vi "3d_display5.vi"() -> ()   [LabVIEW 2009]
doc: "This example demonstrates some fundamental concepts for the 3D picture control. Concepts covered include:\n\n-Object creation\n-Texturing\n-Object movement\n-Object hierarchy"
uses:
  labWOOOO/wiimotestate.ctl
  labWOOOO/wiimoteState(IR).ctl
  <vilib>/Utility/miscctls.llb/LVRectTypeDef.ctl
  C:/Documents and Settings/pbooth/My Documents/labWOOOO/WiimoteLib.dll
  <vilib>/picture/3D Picture Control/NI_3D Picture Control.lvlib
  <vilib>/Analysis/NI_AALBase.lvlib
panel:
  out "angle":dbl
  in  "Y":dbl
  out "trackerino":bool
  out "Blinky":bool
  out "angle 3":sgl
  out "Value 2":sgl
  out "Value":sgl
  out "Cluster":cluster{"Wiimote State":T1, "IRState":T2} {"IRState"."Mode" items=["Off"=0, "Basic"=1, "Extended"=3, "Full"=5]}
  out "raw pitot":dbl
  in  "Calibrate pitot":bool
  in  "voltage offset":dbl=2.5
  in  "velocity scale":dbl=100000.0
  in  "Set Start Time (s)":dbl
  in  "X":dbl
  in  "Z":dbl
  in  "Calibrate Z":bool
  in  "Calibrate Y":bool
  in  "Calibrate X":bool
  out "angle 2":dbl
  out "angle 1":dbl
  out "X mean acceleration":dbl format="%0.4f"
  out "Y mean acceleration":dbl format="%0.4f"
  out "X mean volts":dbl format="%0.4f"
  out "Y mean volts":dbl format="%0.4f"
  out "Z mean acceleration":dbl format="%0.4f"
  out "Z mean volts":dbl format="%0.4f"
  in  "z gain":dbl=5.0
  in  "z offset":dbl=1.25
  in  "y gain":dbl=5.0
  in  "y offset":dbl=1.25
  in  "x gain":dbl=5.0
  in  "x offset":dbl=1.25
  in  "Render Dest":enum16{"Scene Window", "Scene Display"}(ring)=enum."Scene Display"
  in  "Camera Controller":enum16{"None", "Spherical", "Flying"}(ring)=enum."Spherical"
  out "Scene Display":refnum<vi>(3d-picture)
  in  "stop":bool
  # "Accelerometers"
  # "Buttons"
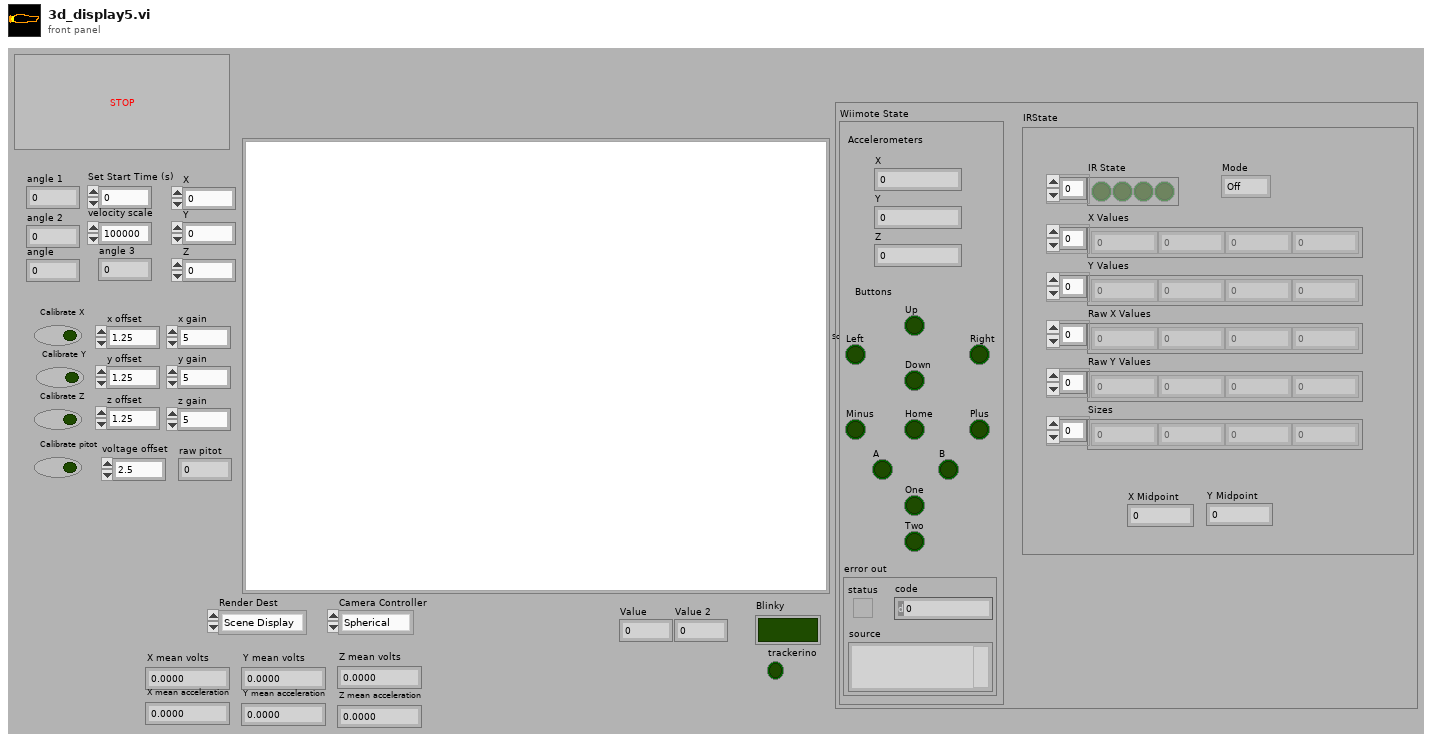
[diagram p1: front panel]
types:
  T1 = typedef "wiimotestate.ctl" = cluster{"X":sgl, "Y":sgl, "Z":sgl, "A":bool, "B":bool, "Down":bool, "Home":bool, "Left":bool, "Minus":bool, "One":bool, "Plus":bool, "Right":bool, "Two":bool, "Up":bool, "error out":errorcluster}
  T2 = typedef "wiimoteState(IR).ctl" = cluster{"Mode":u8, "IR State":bool[], "X Values":sgl[], "Y Values":sgl[], "Raw X Values":i32[], "Raw Y Values":i32[], "Sizes":i32[], "X Midpoint":sgl, "Y Midpoint":sgl}
  T3 = enum16{"As a Decal", "With Modulation", "With Blending", "As a replacement"}
  T4 = typedef "LVRectTypeDef.ctl" = cluster{"Left":i16, "Top":i16, "Right":i16, "Bottom":i16}
  T5 = enum16{"Open", "Minimized", "Maximized", "Hidden"}
  T6 = typedef "imagedata.ctl" = cluster{"image type":i32, "image depth":i32, "image":u8[], "mask":u8[], "colors":u32[], "Rectangle":cluster{"left":i16, "top":i16, "right":i16, "bottom":i16}}
  T7 = cluster{"Mode":u8, "IR State":bool[], "X Values":sgl[], "Y Values":sgl[], "Raw X Values":i32[], "Raw Y Values":i32[], "Sizes":i32[], "X Midpoint":sgl, "Y Midpoint":sgl}
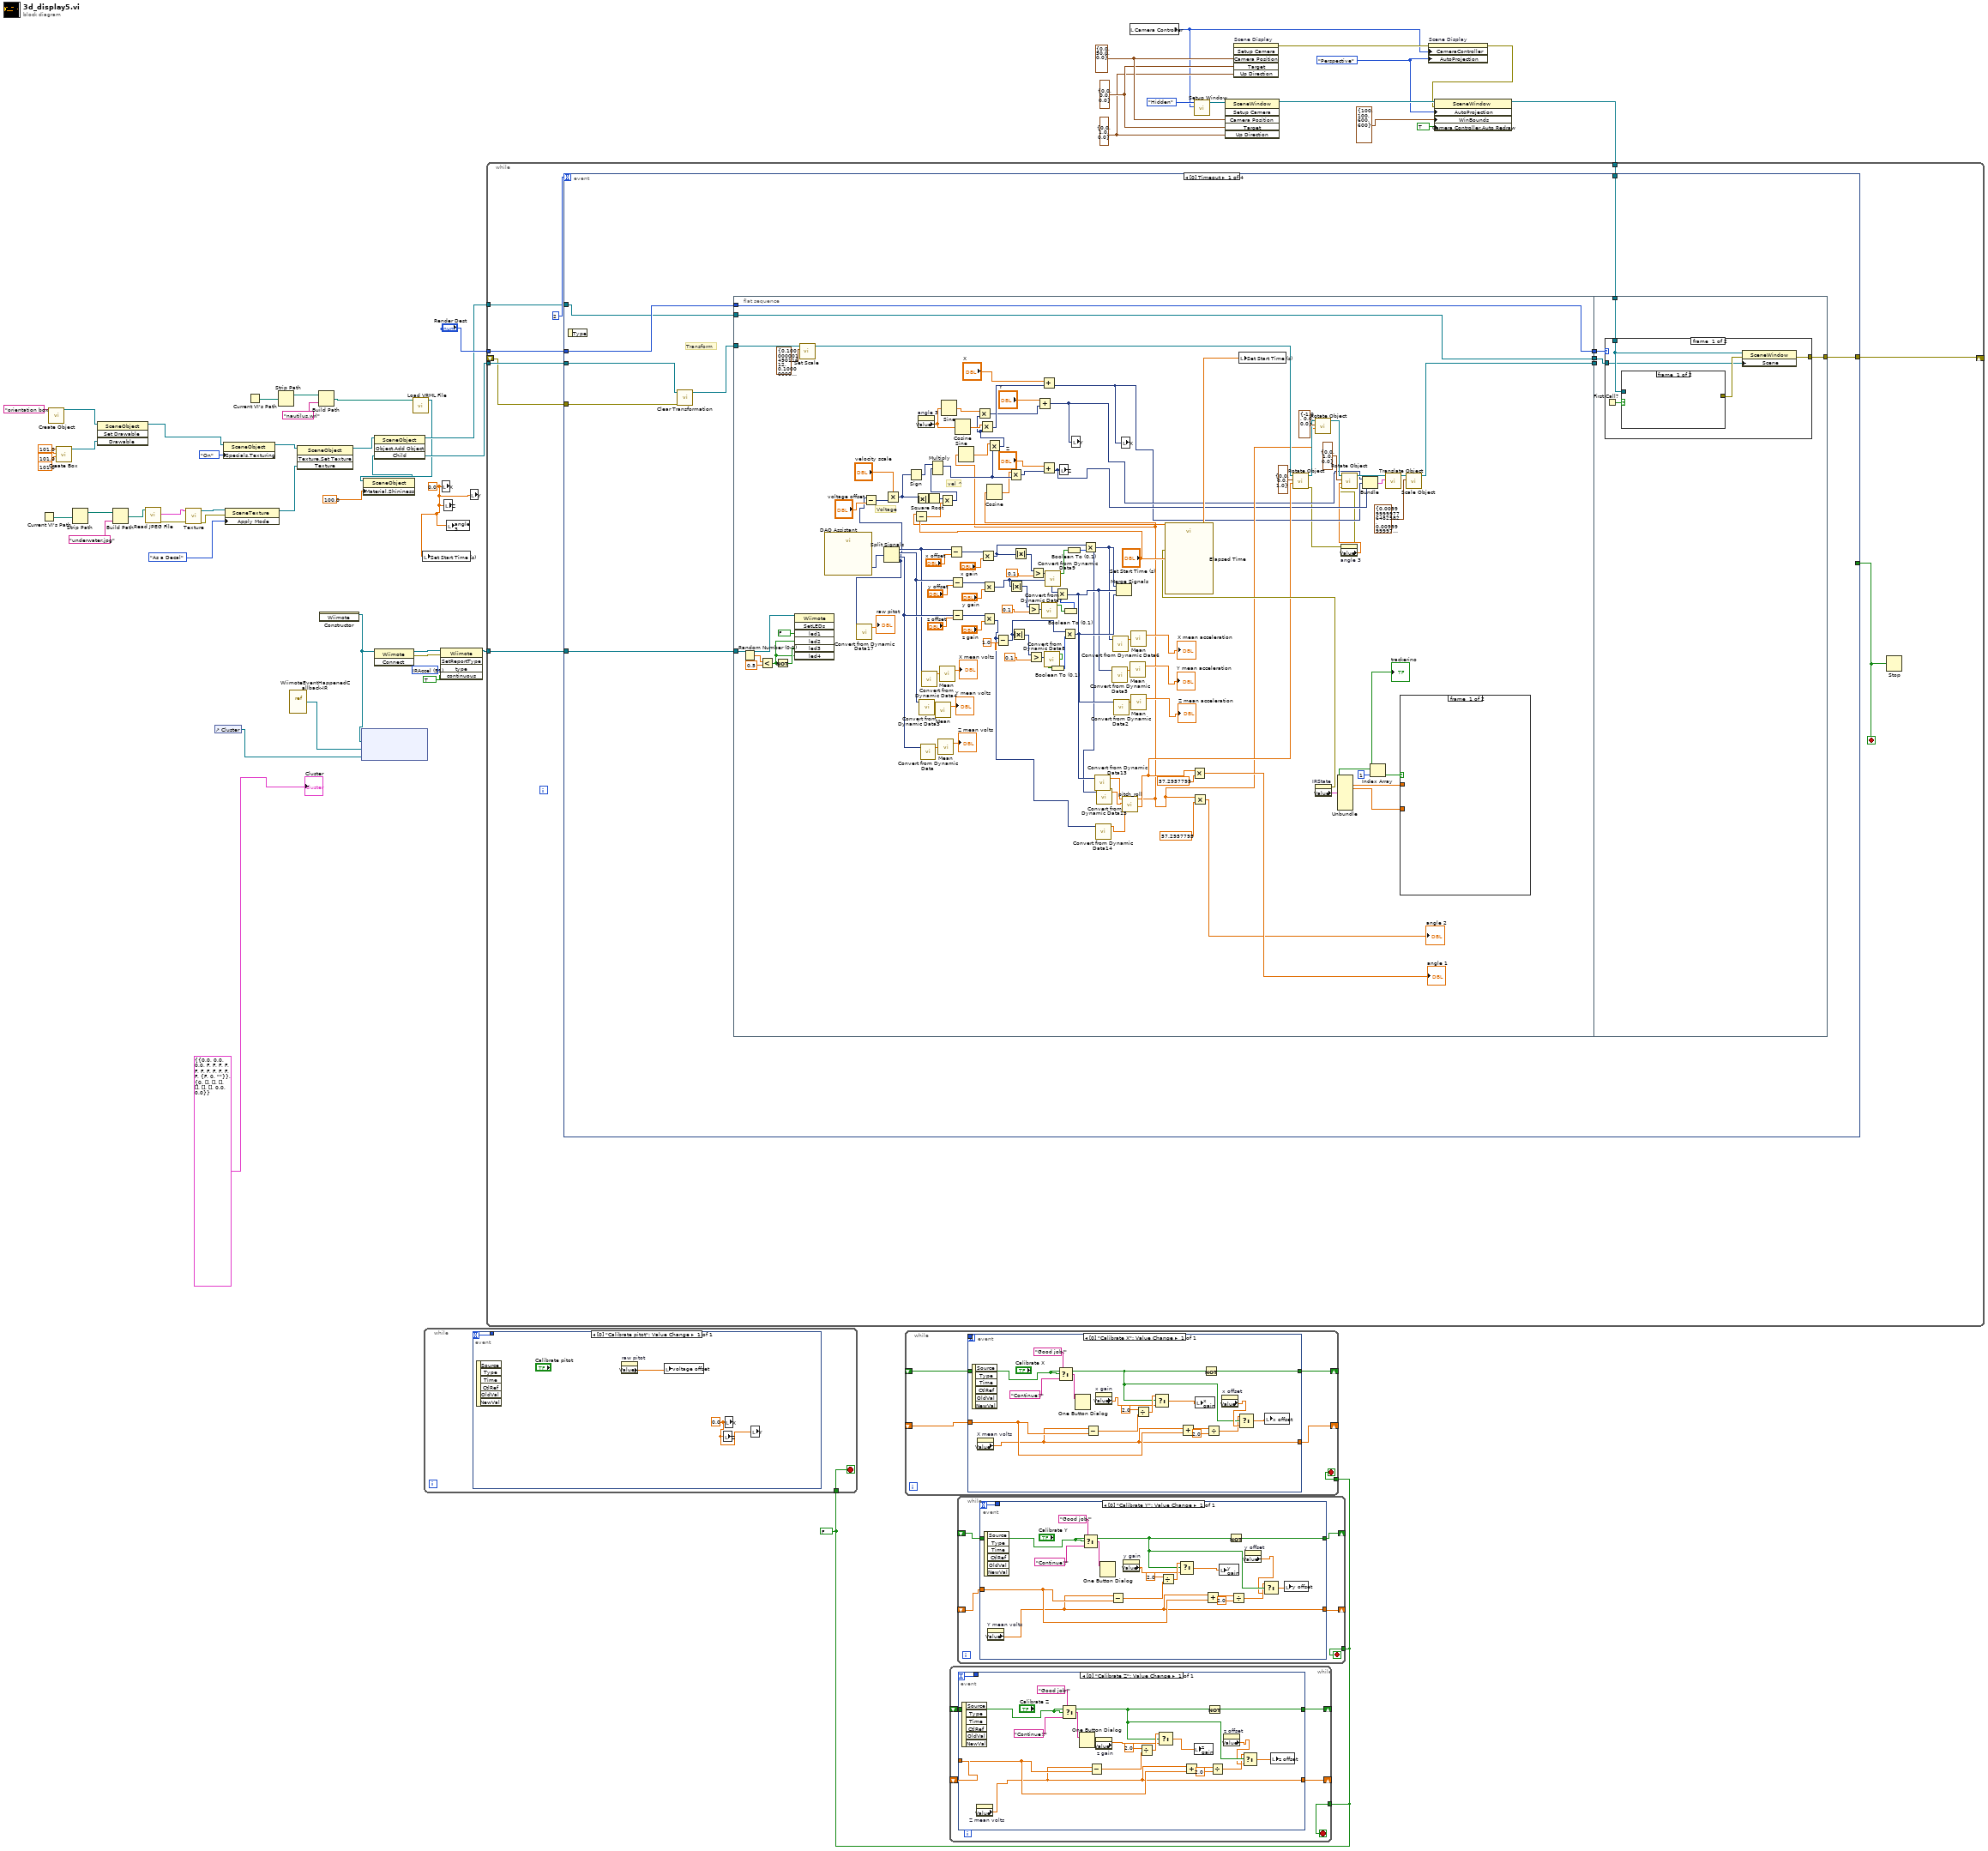
[diagram p0: block diagram]
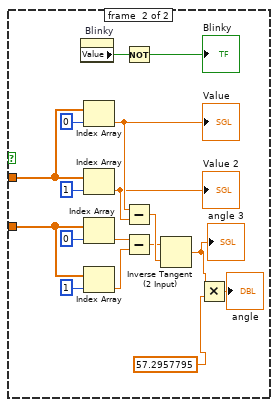
[diagram p2: hidden frame]
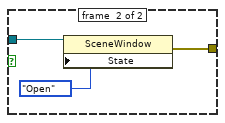
[diagram p3: hidden frame]
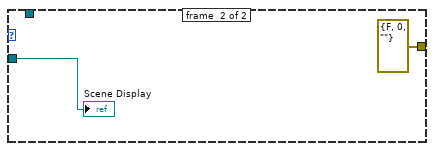
[diagram p4: hidden frame]
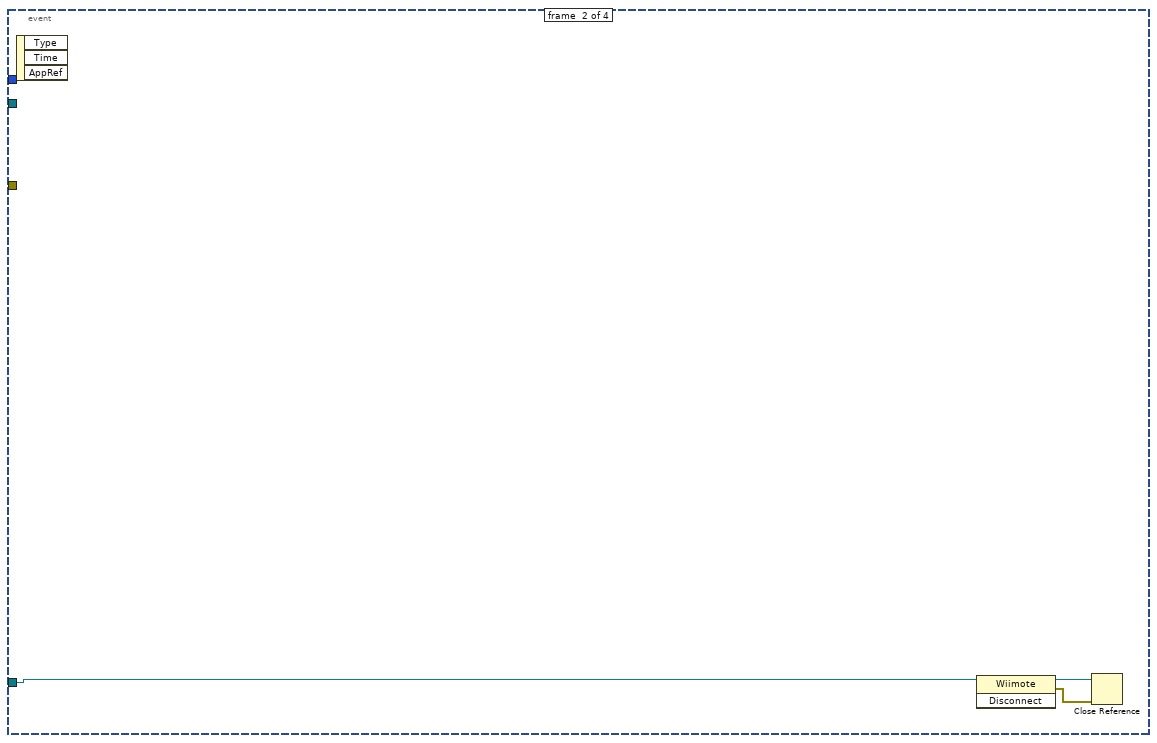
[diagram p5: hidden frame]
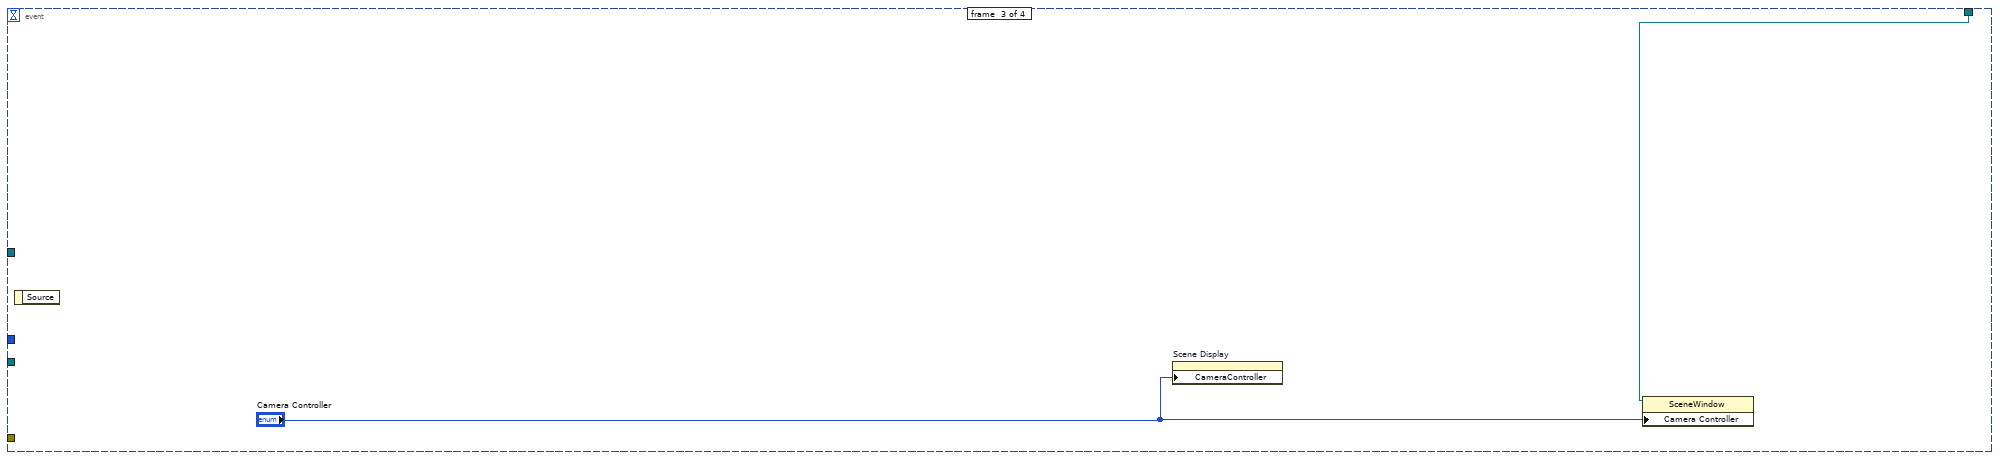
[diagram p6: hidden frame]
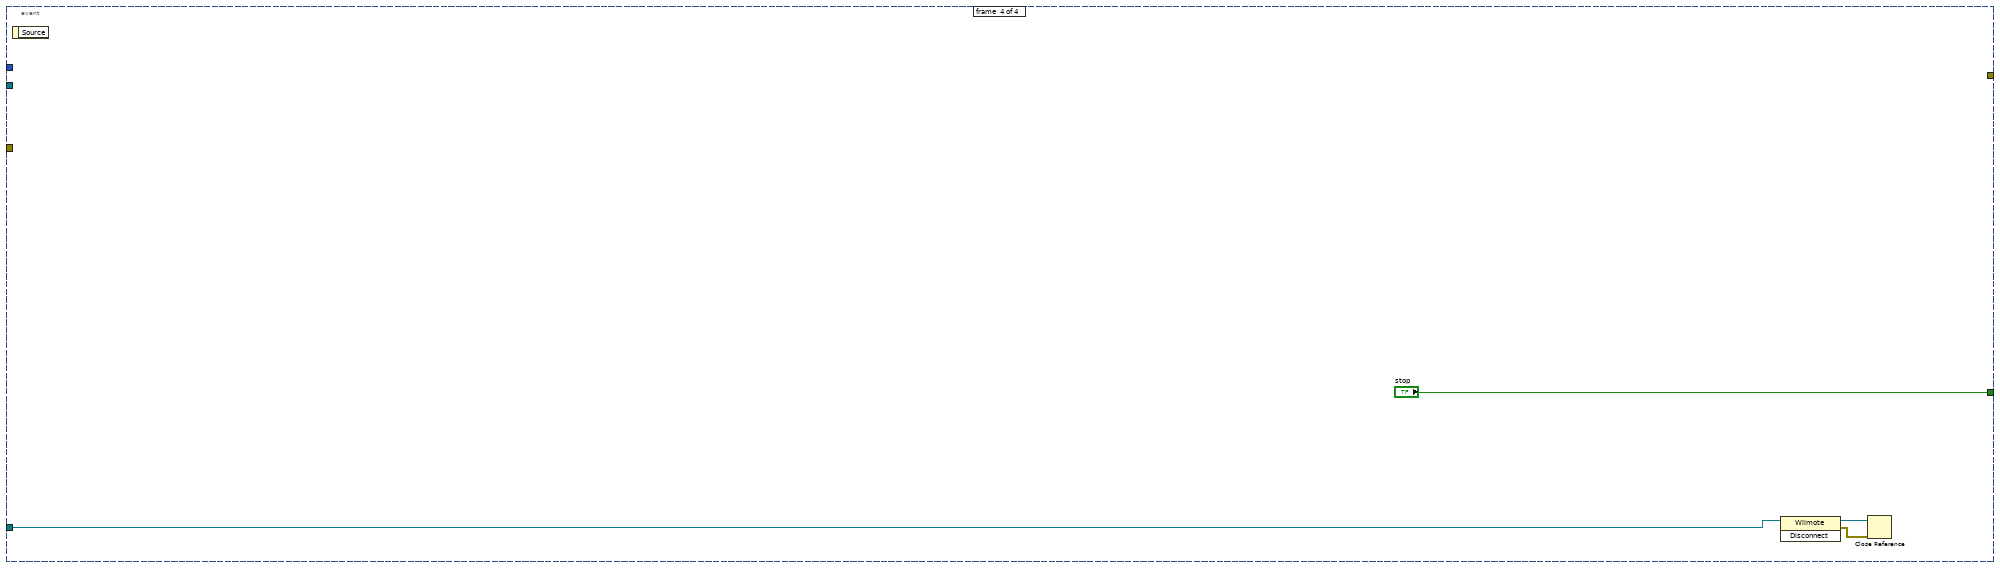
[diagram p7: hidden frame]
diagram:
  w7 = FALSE
  w32 = u8 51 items=["Status"=32, "ReadData"=33, "Buttons"=48, "ButtonsAccel"=49, "IRAccel"=51, "ButtonsExtension"=52, "ExtensionAccel"=53, "IRExtensionAccel"=55] ("type")
  w9 = 0.0 ("X")
  w48 = enum16{"None", "Perspective", "Orthographic"}."Perspective" ("Auto Projection Mode")
  w51 = cluster{"X":sgl, "Y":sgl, "Z":sgl} {"X"=0.0, "Y"=1.0, "Z"=0.0} ("Up Direction")
  w52 = cluster{"X":sgl, "Y":sgl, "Z":sgl} {"X"=0.0, "Y"=0.0, "Z"=0.0} ("Target")
  w53 = cluster{"X":sgl, "Y":sgl, "Z":sgl} {"X"=0.0, "Y"=50.0, "Z"=0.0} ("Camera Position")
  n1 = Current VI's Path() -> (path=w22:path)
  n2 = call <vilib>:"Create Object.vi"("Name"="orientation box") -> ("Scene:New Object"=w26:refnum<vi>)  [unwired: 9 in, 1 out]
  n3 = call <vilib>:"Create Box.vi"("Length Z"=sgl 101.0, "Length Y"=sgl 101.0, "Length X"=sgl 101.0) -> ("New Box Refnum"=w24:refnum<vi>)  [unwired: 7 in, 1 out]
  n4 = Strip Path(path=w22) -> (stripped path=w23:path)  [unwired: 1 out]
  n5 = invoke class="SceneObject" method="Set Drawable"(reference=w26, "Drawable"=w24) -> (reference out=w15:refnum<vi>)  [unwired: 2 in, 3 out]
  n6 = Build Path(base path=w23, name or relative path="underwater.jpg") -> (appended path=w20:path)
  n7 = call <vilib>:"Read JPEG File.vi"("path to JPEG file"=w20) -> ("error out"=w13:errorcluster, "image data"=w14:T6)  [unwired: 8 in, 1 out]
  n8 = call <vilib>:"Texture.vi"("error in (no error)"=w13, "Image"=w14) -> ("error out"=w12:errorcluster, "New Texture Refnum"=w11:refnum<vi>)  [unwired: 8 in]
  n9 = control-ref of="Cluster"() -> (w35:refnum<vi>)
  n10 = property class="SceneObject"(reference=w15, "Specials.Texturing"=enum16{"Inherit Value", "Off", "On"}."On" ("Specials:Texturing")) -> (reference out=w16:refnum<vi>)  [unwired: 1 in, 1 out]
  n11 = property class="SceneTexture"(reference=w11, error in=w12, "Apply Mode"=T3."As a Decal") -> (reference out=w18:refnum<vi>)  [unwired: 1 out]
  n12 = Current VI's Path() -> (path=w41:path)
  n13 = Strip Path(path=w41) -> (stripped path=w42:path)  [unwired: 1 out]
  n14 = vi-ref "WiimoteEventHappenedCallback-IR.vi"() -> ("vi reference"=w38:refnum<vi>)
  n15 = invoke class="SceneObject" method="Texture.Set Texture"(reference=w16, "Texture"=w18) -> (reference out=w6:refnum<vi>)  [unwired: 2 in, 3 out]
  n16 = Build Path(base path=w42, name or relative path="nautilus.wrl") -> (appended path=w39:path)
  n17 = constructor class="Wiimote"() -> (reference out=w37:refnum<k24>)  [unwired: 3 in, 2 out]
  n18 = node(w37, w38, w35) -> ()  [unwired: 2 in, 2 out]
  n19 = invoke class="Wiimote" method="Connect"(reference=w37) -> (reference out=w34:refnum<k24>, error out=w33:errorcluster)  [unwired: 2 in, 1 out]
  n20 = call <vilib>:"Load VRML File.vi"("Path"=w39) -> ("Scene:Read Scene File"=w2:refnum<vi>)  [unwired: 9 in, 1 out]
  n21 = property class="SceneObject"(reference=w2, "Material.Shininess"=sgl 100.0 ("Material:Shininess")) -> (reference out=w1:refnum<vi>)  [unwired: 1 in, 1 out]
  n22 = invoke class="SceneObject" method="Object.Add Object"(reference=w6, "Child"=w1) -> (reference out=w4:refnum<vi>, "Child"=w5:refnum<vi>)  [unwired: 2 in, 2 out]
  n23 = local write "Set Start Time (s)"(w9) -> ()
  n24 = while {
    tunnel: w7 -> [w55]
    stop <- w55 stop-if-true
    n25 = event shown="[0] \"Calibrate pitot\": Value Change" {
      selector: _ -> [_]
      dyn-events: _ -> [_]
      timeout: _ -> [w58]
      tunnel: [w58] -> _
      event [0] "Calibrate pitot": Value Change {
        w56 = 0.0 ("X")
        n26 = event-data() -> ()  [unwired: 1 in, 6 out]
        n27 = property on="raw pitot" class="DigNum (strict)"() -> ("Value"=w57:dbl)  [unwired: 2 in, 2 out]
        n28 = local write "voltage offset"(w57) -> ()
        n29 = local write "Z"(w56) -> ()
        n30 = local write "X"(w56) -> ()
        n31 = local write "Y"(w56) -> ()
      }
    }
  }
  n32 = invoke class="Wiimote" method="SetReportType"(reference=w34, error in=w33, "type"=w32, "continuous"=TRUE) -> (reference out=w8:refnum<k24>)  [unwired: 1 in, 4 out]
  n33 = local write "X"(w9) -> ()
  n34 = local write "Z"(w9) -> ()
  n35 = local write "angle 3"(w9) -> ()
  n36 = local write "Y"(w9) -> ()
  n37 = while {
    shift-right: [w62] -> _
    shift-left: _ -> [w63]
    shift-right: [w61] -> _
    shift-left: _ -> [w60]
    tunnel: w7 -> [w59]
    stop <- w59 stop-if-true
    n38 = event shown="[0] \"Calibrate X\": Value Change" {
      selector: _ -> [_]
      dyn-events: _ -> [_]
      timeout: _ -> [w81]
      tunnel: [w81] -> _
      tunnel: w63 -> [w69]
      tunnel: [w77] -> w62
      tunnel: [w64] -> w61
      tunnel: w60 -> [w68]
      event [0] "Calibrate X": Value Change {
        n39 = event-data() -> ()  [unwired: 1 in, 6 out]
        n40 = property on="X mean volts" class="DigNum (strict)"() -> ("Value"=w64:dbl)  [unwired: 2 in, 2 out]
        n41 = Select(t="Good job!" ("message"), s=w69, f="Continue!!" ("message")) -> (s? t:f=w80:string)
        n42 = One Button Dialog(message=w80) -> ()  [unwired: 1 in, 1 out]
        n43 = Subtract(x=w64, y=w68) -> (x-y=w75:dbl)
        n44 = property on="x gain" class="DigNum (strict)"() -> ("Value"=w73:dbl)  [unwired: 2 in, 2 out]
        n45 = Divide(x=2.0, y=w75) -> (x/y=w74:dbl)
        n46 = Select(t=w74, s=w69, f=w73) -> (s? t:f=w72:dbl)
        n47 = Add(x=w64, y=w68) -> (x+y=w66:dbl)
        n48 = local write "x gain"(w72) -> ()
        n49 = Not(x=w69) -> (.not. x?=w77:bool)
        n50 = Divide(x=w66, y=2.0) -> (x/y=w65:dbl)
        n51 = property on="x offset" class="DigNum (strict)"() -> ("Value"=w70:dbl)  [unwired: 2 in, 2 out]
        n52 = Select(t=w65, s=w69, f=w70) -> (s? t:f=w71:dbl)
        n53 = local write "x offset"(w71) -> ()
      }
    }
  }
  n54 = while {
    shift-right: [w84] -> _
    shift-left: _ -> [w83]
    shift-right: [w86] -> _
    shift-left: _ -> [w85]
    tunnel: w7 -> [w82]
    stop <- w82 stop-if-true
    n55 = event shown="[0] \"Calibrate Z\": Value Change" {
      selector: _ -> [_]
      dyn-events: _ -> [_]
      timeout: _ -> [w104]
      tunnel: [w104] -> _
      tunnel: w85 -> [w96]
      tunnel: [w100] -> w86
      tunnel: [w87] -> w84
      tunnel: w83 -> [w95]
      event [0] "Calibrate Z": Value Change {
        n56 = event-data() -> ()  [unwired: 1 in, 6 out]
        n57 = property on="Z mean volts" class="DigNum (strict)"() -> ("Value"=w87:dbl)  [unwired: 2 in, 2 out]
        n58 = Select(t="Good job!" ("message"), s=w96, f="Continue!!" ("message")) -> (s? t:f=w103:string)
        n59 = One Button Dialog(message=w103) -> ()  [unwired: 1 in, 1 out]
        n60 = Subtract(x=w87, y=w95) -> (x-y=w98:dbl)
        n61 = property on="z gain" class="DigNum (strict)"() -> ("Value"=w90:dbl)  [unwired: 2 in, 2 out]
        n62 = Divide(x=2.0, y=w98) -> (x/y=w97:dbl)
        n63 = Select(t=w97, s=w96, f=w90) -> (s? t:f=w88:dbl)
        n64 = Add(x=w87, y=w95) -> (x+y=w93:dbl)
        n65 = local write "z gain"(w88) -> ()
        n66 = Not(x=w96) -> (.not. x?=w100:bool)
        n67 = Divide(x=w93, y=2.0) -> (x/y=w92:dbl)
        n68 = property on="z offset" class="DigNum (strict)"() -> ("Value"=w89:dbl)  [unwired: 2 in, 2 out]
        n69 = Select(t=w92, s=w96, f=w89) -> (s? t:f=w91:dbl)
        n70 = local write "z offset"(w91) -> ()
      }
    }
  }
  n71 = while {
    shift-right: [w109] -> _
    shift-left: _ -> [w108]
    shift-right: [w106] -> _
    shift-left: _ -> [w107]
    tunnel: w7 -> [w105]
    stop <- w105 stop-if-true
    n72 = event shown="[0] \"Calibrate Y\": Value Change" {
      selector: _ -> [_]
      dyn-events: _ -> [_]
      timeout: _ -> [w127]
      tunnel: [w127] -> _
      tunnel: w108 -> [w119]
      tunnel: [w123] -> w109
      tunnel: [w110] -> w106
      tunnel: w107 -> [w118]
      event [0] "Calibrate Y": Value Change {
        n73 = event-data() -> ()  [unwired: 1 in, 6 out]
        n74 = property on="Y mean volts" class="DigNum (strict)"() -> ("Value"=w110:dbl)  [unwired: 2 in, 2 out]
        n75 = Select(t="Good job!" ("message"), s=w119, f="Continue!!" ("message")) -> (s? t:f=w126:string)
        n76 = One Button Dialog(message=w126) -> ()  [unwired: 1 in, 1 out]
        n77 = Subtract(x=w110, y=w118) -> (x-y=w121:dbl)
        n78 = property on="y gain" class="DigNum (strict)"() -> ("Value"=w114:dbl)  [unwired: 2 in, 2 out]
        n79 = Divide(x=2.0, y=w121) -> (x/y=w120:dbl)
        n80 = Select(t=w120, s=w119, f=w114) -> (s? t:f=w113:dbl)
        n81 = Add(x=w110, y=w118) -> (x+y=w116:dbl)
        n82 = local write "y gain"(w113) -> ()
        n83 = Not(x=w119) -> (.not. x?=w123:bool)
        n84 = Divide(x=w116, y=2.0) -> (x/y=w115:dbl)
        n85 = property on="y offset" class="DigNum (strict)"() -> ("Value"=w112:dbl)  [unwired: 2 in, 2 out]
        n86 = Select(t=w115, s=w119, f=w112) -> (s? t:f=w111:dbl)
        n87 = local write "y offset"(w111) -> ()
      }
    }
  }
  n88 = local read "Camera Controller"() -> (w45:enum16{"None", "Spherical", "Flying"})
  n89 = call <vilib>:"Setup Window.vi"("Camera Controller"=w45, "Window State"=T5."Hidden") -> ("New Window Refnum"=w47:refnum<vi>)  [unwired: 1 in, 8 out]
  n90 = invoke class="SceneWindow" method="Setup Camera"(reference=w47, "Camera Position"=w53, "Target"=w52, "Up Direction"=w51) -> (reference out=w54:refnum<vi>)  [unwired: 2 in, 5 out]
  n91 = invoke on="Scene Display" class="SceneGraphDisp (strict)" method="Setup Camera"("Camera Position"=w53, "Target"=w52, "Up Direction"=w51) -> (error out=w50:errorcluster)  [unwired: 3 in, 5 out]
  n92 = property on="Scene Display" class="SceneGraphDisp (strict)"(error in=w50, "CameraController"=w45, "AutoProjection"=w48) -> (error out=w49:errorcluster)  [unwired: 1 in, 1 out]
  n93 = property class="SceneWindow"(reference=w54, error in=w49, "AutoProjection"=w48, "WinBounds"=T4 {"Left"=100, "Top"=100, "Right"=600, "Bottom"=600} ("Window Bounds"), "Camera Controller.Auto Redraw"=TRUE ("Camera Controller:Auto Redraw")) -> (reference out=w30:refnum<vi>)  [unwired: 1 out]
  n94 = while {
    tunnel: w30 -> [w136]
    tunnel: w5 -> [w135]
    tunnel: w8 -> [w134]
    tunnel: "Render Dest" -> [w131]
    shift-right: [w130] -> _
    shift-left: _ -> [w129]
    tunnel: w4 -> [w128]
    stop <- w132 stop-if-true
    n95 = event shown="[0] Timeout" {
      selector: _ -> [_ _ _ _]
      dyn-events: _ -> [_ _ _ _]
      timeout: 2 -> [_ _ _ _]
      tunnel: w136 -> [w141 _ w300 _]
      tunnel: w135 -> [w144 _ _ _]
      tunnel: [_ _ _ "stop"] -> w132
      tunnel: w131 -> [w145 _ _ _]
      tunnel: w134 -> [w142 w296 _ w302]
      tunnel: [w140 _ _ _] -> w130
      tunnel: w129 -> [w139 _ _ _]
      tunnel: w128 -> [w138 _ _ _]
      event #0 {
        # "Transform"
        n96 = event-data() -> ()  [unwired: 2 out]
        n97 = call <vilib>:"Clear Transformation.vi"("error in (no error)"=w139, "Object Refnum In"=w144) -> ("Object Refnum Out"=w147:refnum<vi>)  [unwired: 9 out]
        n98 = flat-sequence {
          tunnel: w147 -> [w199]
          tunnel: [w264] -> w146
          tunnel: w145 -> [w264]
          tunnel: [w161] -> w143
          tunnel: w142 -> [w184]
          tunnel: w138 -> [w158]
          tunnel: [w158] -> w137
          tunnel: w141 -> [w285]
          tunnel: w146 -> [w284]
          tunnel: w143 -> [_]
          tunnel: [w283] -> w140
          tunnel: w137 -> [w282]
          frame #0 {
            # "vel ^"
            # "Voltage"
            n99 = Random Number (0-1)() -> (number: 0 to 1=w182:dbl)
            n100 = Less?(x=w182, y=0.5) -> (x < y?=w179:bool)
            n101 = Not(x=w179) -> (.not. x?=w180:bool)
            n102 = invoke class="Wiimote" method="SetLEDs"(reference=w184, "led1"=FALSE, "led2"=w179, "led3"=w180, "led4"=w179) -> ()  [unwired: 2 in, 7 out]
            n103 = call <vilib>:"Set Scale.vi"("Scale"=cluster{"X":sgl, "Y":sgl, "Z":sgl} {"X"=0.1, "Y"=0.1, "Z"=0.1}, "Scene Object"=w199) -> ("Scaled Object"=w162:refnum<vi>)  [unwired: 8 in, 1 out]
            n104 = call "DAQ Assistant"() -> ("data"=w214:dynamicdata)  [unwired: 17 in, 2 out]
            n105 = Split Signals(w214) -> (w245:dynamicdata, w247:dynamicdata, w250:dynamicdata, w190:dynamicdata)  [unwired: 4 in]
            n106 = call "Convert from Dynamic Data17"("Dynamic Data Type"=w190) -> ("Scalar"=→"raw pitot":dbl)  [unwired: 3 in]
            n107 = Subtract(x=w190, y="voltage offset") -> (x-y=w212:dynamicdata)
            n108 = Multiply(x="velocity scale", y=w212) -> (x*y=w157:dynamicdata)
            n109 = Sign(1:w157) -> (0:w156:dynamicdata)
            n110 = Absolute Value(x=w157) -> (abs(x)=w203:dynamicdata)
            n111 = property on="angle 3" class="DigNum (strict)"() -> ("Value"=w168:sgl)  [unwired: 2 in, 2 out]
            n112 = call "Convert from Dynamic Data3"("Dynamic Data Type"=w247) -> ("Array"=w246:dbl[])  [unwired: 3 in]
            n113 = call "Convert from Dynamic Data"("Dynamic Data Type"=w250) -> ("Array"=w252:dbl[])  [unwired: 3 in]
            n114 = call "Convert from Dynamic Data4"("Dynamic Data Type"=w245) -> ("Array"=w244:dbl[])  [unwired: 3 in]
            n115 = Square Root(x=w203) -> (sqrt(x)=w202:dynamicdata)
            n116 = call <vilib>:"Mean.vi"("X"=w246) -> ("mean"=→"Y mean volts":dbl)  [unwired: 1 out]
            n117 = call <vilib>:"Mean.vi"("X"=w252) -> ("mean"=→"Z mean volts":dbl)  [unwired: 1 out]
            n118 = call <vilib>:"Mean.vi"("X"=w244) -> ("mean"=→"X mean volts":dbl)  [unwired: 1 out]
            n119 = Sine(x=w168) -> (sin(x)=w154:sgl)
            n120 = Subtract(x=w245, y="x offset") -> (x-y=w261:dynamicdata)
            n121 = Subtract(x=w247, y="y offset") -> (x-y=w257:dynamicdata)
            n122 = Subtract(x=w250, y="z offset") -> (x-y=w239:dynamicdata)
            n123 = Cosine(x=w168) -> (cos(x)=w167:sgl)
            n124 = Multiply(x=w261, y="x gain") -> (x*y=w220:dynamicdata)
            n125 = Multiply(x=w257, y="y gain") -> (x*y=w238:dynamicdata)
            n126 = Multiply(x=w239, y="z gain") -> (x*y=w193:dynamicdata)
            n127 = Subtract(x=w193, y=1.0) -> (x-y=w226:dynamicdata)
            n128 = Absolute Value(x=w238) -> (abs(x)=w237:dynamicdata)
            n129 = Absolute Value(x=w226) -> (abs(x)=w232:dynamicdata)
            n130 = Absolute Value(x=w220) -> (abs(x)=w225:dynamicdata)
            n131 = Greater?(x=w237, y=0.1) -> (0:w234:dynamicdata)
            n132 = Greater?(x=w232, y=0.1) -> (0:w230:dynamicdata)
            n133 = Greater?(x=w225, y=0.1) -> (0:w222:dynamicdata)
            n134 = call "Convert from Dynamic Data7"("Dynamic Data Type"=w234) -> ("Scalar"=w233:bool)  [unwired: 3 in]
            n135 = call "Convert from Dynamic Data8"("Dynamic Data Type"=w230) -> ("Scalar"=w229:bool)  [unwired: 3 in]
            n136 = call "Convert from Dynamic Data9"("Dynamic Data Type"=w222) -> ("Scalar"=w221:bool)  [unwired: 3 in]
            n137 = Boolean To (0,1)(Boolean=w229) -> (0, 1=w228:i16)
            n138 = Boolean To (0,1)(Boolean=w233) -> (0, 1=w235:i16)
            n139 = Multiply(x=w238, y=w235) -> (x*y=w195:dynamicdata)
            n140 = Multiply(x=w226, y=w228) -> (x*y=w209:dynamicdata)
            n141 = Boolean To (0,1)(Boolean=w221) -> (0, 1=w223:i16)
            n142 = Multiply(x=w220, y=w223) -> (x*y=w194:dynamicdata)
            n143 = call "Convert from Dynamic Data13"("Dynamic Data Type"=w195) -> ("Scalar"=w187:dbl)  [unwired: 3 in]
            n144 = call "Convert from Dynamic Data14"("Dynamic Data Type"=w193) -> ("Scalar"=w186:dbl)  [unwired: 3 in]
            n145 = call "Convert from Dynamic Data15"("Dynamic Data Type"=w194) -> ("Scalar"=w185:dbl)  [unwired: 3 in]
            n146 = call "Convert from Dynamic Data5"("Dynamic Data Type"=w195) -> ("Array"=w241:dbl[])  [unwired: 3 in]
            n147 = call "Convert from Dynamic Data6"("Dynamic Data Type"=w194) -> ("Array"=w240:dbl[])  [unwired: 3 in]
            n148 = call "Convert from Dynamic Data2"("Dynamic Data Type"=w209) -> ("Array"=w251:dbl[])  [unwired: 3 in]
            n149 = Merge Signals(w194, w195, w209) -> ()  [unwired: 1 out]
            n150 = call "pitch_roll.vi"("Az"=w186, "Ay"=w185, "Ax"=w187) -> ("Pitch"=w160:dbl, "Roll"=w159:dbl)  [unwired: 7 in]
            n151 = Sine(x=w159) -> (sin(x)=w155:dbl)
            n152 = Cosine(x=w159) -> (cos(x)=w197:dbl)
            n153 = call <vilib>:"Mean.vi"("X"=w241) -> ("mean"=→"Y mean acceleration":dbl)  [unwired: 1 out]
            n154 = call <vilib>:"Mean.vi"("X"=w240) -> ("mean"=→"X mean acceleration":dbl)  [unwired: 1 out]
            n155 = call <vilib>:"Mean.vi"("X"=w251) -> ("mean"=→"Z mean acceleration":dbl)  [unwired: 1 out]
            n156 = Multiply(x=w160, y=57.2957795) -> (x*y=→"angle 1":dbl)
            n157 = Multiply(x=w159, y=57.2957795) -> (x*y=→"angle 2":dbl)
            n158 = call <vilib>:"Rotate Object.vi"("Angle"=w160, "Axis"=cluster{"X":sgl, "Y":sgl, "Z":sgl} {"X"=0.0, "Y"=0.0, "Z"=1.0}, "Scene.Object In"=w162) -> ("error out"=w148:errorcluster, "Scene.Object Out"=w192:refnum<vi>)  [unwired: 7 in]
            n159 = call <vilib>:"Rotate Object.vi"("Angle"=w159, "Axis"=cluster{"X":sgl, "Y":sgl, "Z":sgl} {"X"=-1.0, "Y"=0.0, "Z"=0.0}, "Scene.Object In"=w192) -> ("Scene.Object Out"=w171:refnum<vi>)  [unwired: 7 in, 1 out]
            n160 = property on="IRState" class="Clust (strict)"() -> (error out=w169:errorcluster, "Value"=w178:T7)  [unwired: 2 in, 1 out]
            n161 = call "Elapsed Time"("error in (no error)"=w169, "Set Start Time (s)"="Set Start Time (s)") -> ("Elapsed Time (s)"=w188:dbl)  [unwired: 10 in, 7 out]
            n162 = Subtract(x=w188, y="Set Start Time (s)") -> (x-y=w204:dbl)
            n163 = Multiply(x=w202, y=w204) -> (x*y=w201:dynamicdata)
            n164 = Multiply(1:w201, 2:w156) -> (0:w200:dynamicdata)  [unwired: 1 in, 1 out]
            n165 = Multiply(x=w155, y=w200) -> (x*y=w166:dynamicdata)
            n166 = Multiply(x=w154, y=w166) -> (x*y=w163:dynamicdata)
            n167 = Multiply(x=w167, y=w166) -> (x*y=w164:dynamicdata)
            n168 = Multiply(x=w197, y=w200) -> (x*y=w208:dynamicdata)
            n169 = Add(x="Y", y=w163) -> (x+y=w152:dynamicdata)
            n170 = Add(x="X", y=w164) -> (x+y=w151:dynamicdata)
            n171 = Add(x="Z", y=w208) -> (x+y=w153:dynamicdata)
            n172 = local write "Z"(w153) -> ()
            n173 = local write "Y"(w152) -> ()
            n174 = local write "X"(w151) -> ()
            n175 = local write "Set Start Time (s)"(w188) -> ()
            n176 = Unbundle(w178) -> ("IR State"=w174:bool[], "X Values"=w177:sgl[], "Y Values"=w176:sgl[])  [unwired: 6 out]
            n177 = property on="angle 3" class="DigNum (strict)"(error in=w148) -> (error out=w149:errorcluster, "Value"=w150:sgl)  [unwired: 1 in, 1 out]
            n178 = call <vilib>:"Rotate Object.vi"("error in (no error)"=w149, "Angle"=w150, "Axis"=cluster{"X":sgl, "Y":sgl, "Z":sgl} {"X"=0.0, "Y"=1.0, "Z"=0.0}, "Scene.Object In"=w171) -> ("Scene.Object Out"=w170:refnum<vi>)  [unwired: 6 in, 1 out]
            n179 = Bundle(w152, w151, w153) -> (w206:cluster{dynamicdata, dynamicdata, dynamicdata})  [unwired: 1 in]
            n180 = Index Array(array=w174, index=1) -> (element=w173:bool)
            "trackerino" <- w173
            n181 = call <vilib>:"Translate Object.vi"("Translation"=w206, "Scene.Object In"=w170) -> ("Scene.Object Out"=w207:refnum<vi>)  [unwired: 8 in, 1 out]
            n182 = case shown="True" w173 {
              tunnel: w177 -> [_ w269]
              tunnel: w176 -> [_ w268]
              frame #0 {
              }
              frame #1 {
                n183 = property on="Blinky" class="Bool (strict)"() -> ("Value"=w271:bool)  [unwired: 2 in, 2 out]
                n184 = Index Array(array=w269, index=0) -> (element=w277:sgl)
                "Value" <- w277
                n185 = Index Array(array=w269, index=1) -> (element=w276:sgl)
                "Value 2" <- w276
                n186 = Index Array(array=w268, index=0) -> (element=w273:sgl)
                n187 = Index Array(array=w268, index=1) -> (element=w272:sgl)
                n188 = Not(x=w271) -> (.not. x?=→"Blinky":bool)
                n189 = Subtract(x=w277, y=w276) -> (x-y=w281:sgl)
                n190 = Subtract(x=w273, y=w272) -> (x-y=w280:sgl)
                n191 = Inverse Tangent (2 Input)(1:w281, 2:w280) -> (0:w267:sgl)
                "angle 3" <- w267
                n192 = Multiply(x=w267, y=57.2957795) -> (x*y=→"angle":dbl)
              }
            }
            n193 = call <vilib>:"Scale Object.vi"("Scale"=cluster{"X":sgl, "Y":sgl, "Z":sgl} {"X"=0.01, "Y"=0.01, "Z"=0.01}, "Scene.Object In"=w207) -> ("Scene.Object Out"=w161:refnum<vi>)  [unwired: 8 in, 1 out]
          }
          frame #1 {
            n194 = case shown="\"Scene Display\"" w284 {
              tunnel: w285 -> [w288 _]
              tunnel: w282 -> [w287 w295]
              tunnel: [w286 errorcluster {"status"=FALSE, "code"=0, "source"=""} ("error out")] -> w283
              frame #0 {
                n195 = First Call?() -> (First Call?: T/F=w289:bool)
                n196 = case shown="True" w289 {
                  tunnel: w288 -> [_ w293]
                  tunnel: [_ w292] -> w290
                  frame #0 {
                  }
                  frame #1 {
                    n197 = property class="SceneWindow"(reference=w293, "State"=T5."Open" ("Window State")) -> (error out=w292:errorcluster)  [unwired: 1 in, 1 out]
                  }
                }
                n198 = property class="SceneWindow"(reference=w288, error in=w290, "Scene"=w287) -> (error out=w286:errorcluster)  [unwired: 1 out]
              }
              frame #1 {
                "Scene Display" <- w295
              }
            }
          }
        }
      }
      event #1 {
        n199 = event-data() -> ()  [unwired: 4 out]
        n200 = invoke class="Wiimote" method="Disconnect"(reference=w296) -> (reference out=w298:refnum<k24>, error out=w297:errorcluster)  [unwired: 2 in, 1 out]
        n201 = Close Reference(reference=w298, error in (no error)=w297) -> ()  [unwired: 1 out]
      }
      event #2 {
        n202 = event-data() -> ()  [unwired: 2 out]
        n203 = property on="Scene Display" class="SceneGraphDisp (strict)"("CameraController"="Camera Controller") -> ()  [unwired: 2 in, 2 out]
        n204 = property class="SceneWindow"(reference=w300, "Camera Controller"="Camera Controller") -> ()  [unwired: 1 in, 2 out]
      }
      event #3 {
        n205 = event-data() -> ()  [unwired: 2 out]
        n206 = invoke class="Wiimote" method="Disconnect"(reference=w302) -> (reference out=w304:refnum<k24>, error out=w303:errorcluster)  [unwired: 2 in, 1 out]
        n207 = Close Reference(reference=w304, error in (no error)=w303) -> ()  [unwired: 1 out]
      }
    }
    n208 = Stop(stop? (T)=w132) -> ()
  }
  "Cluster" <- cluster{"Wiimote State":T1, "IRState":T2} {"Wiimote State"={"X"=0.0, "Y"=0.0, "Z"=0.0, "A"=FALSE, "B"=FALSE, "Down"=FALSE, "Home"=FALSE, "Left"=FALSE, "Minus"=FALSE, "One"=FALSE, "Plus"=FALSE, "Right"=FALSE, "Two"=FALSE, "Up"=FALSE, "error out"={"status"=FALSE, "code"=0, "source"=""}}, "IRState"={"Mode"=0, "IR State"=[], "X Values"=[], "Y Values"=[], "Raw X Values"=[], "Raw Y Values"=[], "Sizes"=[], "X Midpoint"=0.0, "Y Midpoint"=0.0}} ("Cluster")
